vi "selfTest.vi"(0 "HGF_DeviceBase":refnum<class "HGF_DeviceBase.lvclass">, 5 "error in (no error)":errorcluster) -> (14 "dup HGF_DeviceBase":refnum<class "HGF_DeviceBase.lvclass">, 16 "passed?":bool, 17 "resultCode":i32, 18 "resultMessage":string, 19 "error out":errorcluster)   [LabVIEW 2014, in "HGF_DeviceBaseClasses.lvlib" / "HGF_DeviceBase.lvclass"]
doc: "This VI runs the instrument's self test routine and returns the test results.\n\n<b>Hint:</b> This is a dynamic dispatch VI to be implemented by child classes."
uses:
  HGF_DeviceBase.lvclass
  HGF_Auxiliary/HGF_Auxiliary.lvlib
  HGF_Auxiliary/ErrorCode.ctl
  HGF_Auxiliary/Severity.ctl
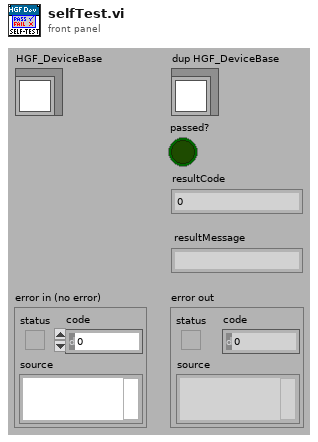
[diagram p1: front panel]
types:
  T1 = typedef "HGF_Auxiliary.lvlib/Severity.ctl" = enum16{"Info", "Warning", "Fault", "Error", "Fatal"}
  T2 = typedef "HGF_Auxiliary.lvlib/ErrorCode.ctl" = enum32{"No error", "Function not supported.", "This VI is for friends only.", "Reference object aready exisits.", "Parameter out of range.", "Not a rendezvous.", "Invalid notifier reference.", "Invalid queue reference.", "Self-Test not supported.", "Reset not supported.", "IDN query not supported.", "Error query not supported.", "Incorrect addressee.", "Object already exists.", "No class name specified", "Driver not supported", "Attribute is not writable"}
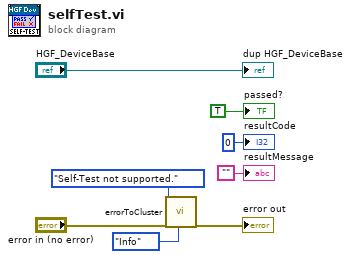
[diagram p0: block diagram]
diagram:
  n1 = call "errorToCluster.vi"("error code"=ErrorCode."Self-Test not supported.", "error in (no error)"="error in (no error)", "severity (Error)"=Severity."Info") -> ("error out"=→"error out":errorcluster)  [unwired: 2 in, 14 out]
  "dup HGF_DeviceBase" <- "HGF_DeviceBase"
  "resultCode" <- 0 ("resultCode")
  "resultMessage" <- ""
  "passed?" <- TRUE ("passed?")
